vi "信号读取.vi"(2 "Boolean":bool) -> (0 "mono 16-bit":dbl[](array[numeric]))   [LabVIEW 2018]
panel:
  out "文件数据":dynamicdata(graph)
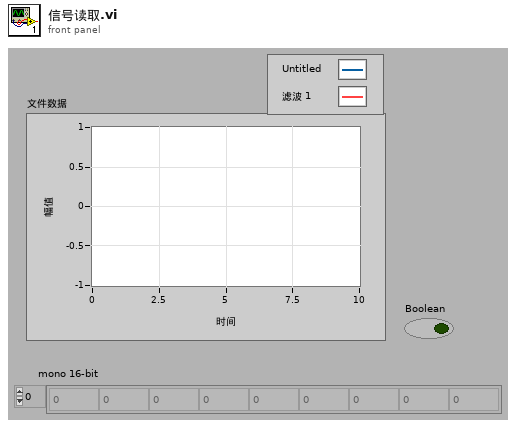
[diagram p1: front panel]
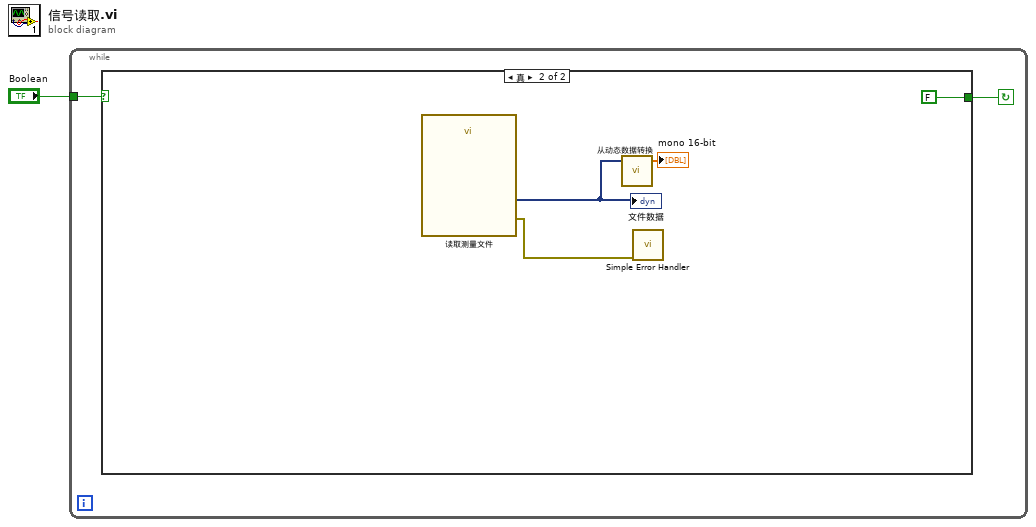
[diagram p0: block diagram]
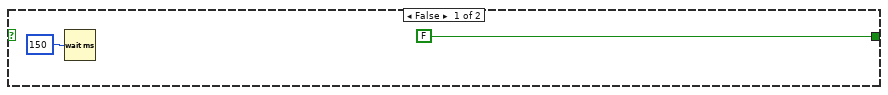
[diagram p2: hidden frame]
diagram:
  n1 = while {
    tunnel: "Boolean" -> [w2]
    stop <- w3 continue-if-true
    n2 = case shown="真" w2 {
      tunnel: [FALSE FALSE] -> w3
      frame False {
        n3 = Wait (ms)(milliseconds to wait=u32 150) -> ()  [unwired: 1 out]
      }
      frame True {
        n4 = call "读取测量文件"() -> ("error out"=w8:errorcluster, "Signals"=w7:dynamicdata)  [unwired: 6 in, 4 out]
        "文件数据" <- w7
        n5 = call "从动态数据转换"("Dynamic Data Type"=w7) -> ("Array"=→"mono 16-bit":dbl[])  [unwired: 3 in]
        n6 = call <vilib>:"Simple Error Handler.vi"("error in (no error)"=w8) -> ()  [unwired: 4 in, 5 out]
      }
    }
  }
